vi "1.6.vi"() -> ()   [LabVIEW 2013]
panel:
  in  "Selector":bool
  out "Temperatura convertida.":dbl
  in  "Temp a convertir":dbl
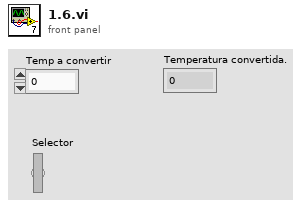
[diagram p1: front panel]
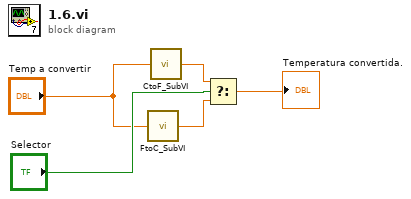
[diagram p0: block diagram]
diagram:
  n1 = call "FtoC_SubVI.vi"("Temperatura a Convertir"="Temp a convertir") -> ("Temperatura Convertida"=w5:dbl)
  n2 = call "CtoF_SubVI.vi"("Temperatura a Convertir"="Temp a convertir") -> ("Temperatura Convertida"=w1:dbl)
  n3 = Select(t=w1, s="Selector", f=w5) -> (s? t:f=→"Temperatura convertida.":dbl)
